vi "Read Glyph.vi"(8 "error in (no error)":errorcluster, 11 "Wait Step UI in":refnum<class "Wait Step UI.lvclass">) -> (0 "error out":errorcluster, 2 "Glyph":string, 3 "Wait Step UI out":refnum<class "Wait Step UI.lvclass">)   [LabVIEW 2015, in "Wait Step UI.lvclass"]
uses:
  Wait Step UI.lvclass
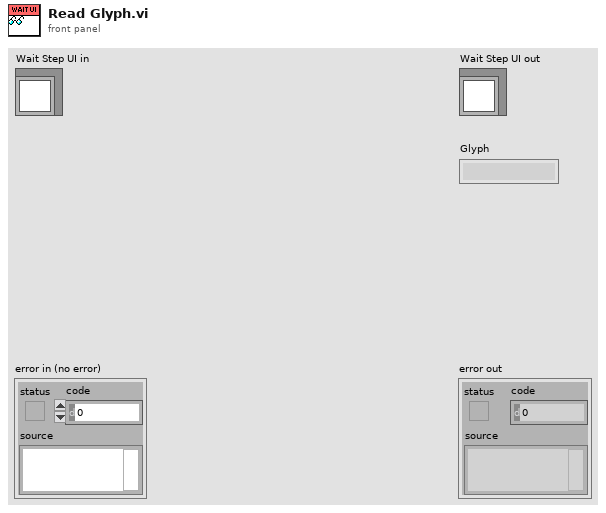
[diagram p1: front panel]
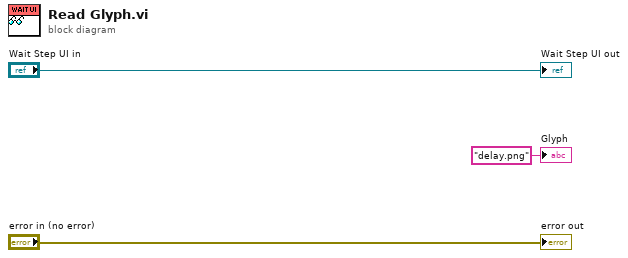
[diagram p0: block diagram]
diagram:
  "error out" <- "error in (no error)"
  "Wait Step UI out" <- "Wait Step UI in"
  "Glyph" <- "delay.png" ("Glyph")
